vi "Making a Dark Sky Forecast Request.vi"() -> ()   [LabVIEW 2017, in "Dark Sky Weather Data for LabVIEW.lvlib"]
doc: "Example shows how to make a Forecast request to the DarkSky API and inteprets the result. A Forecast request returns the current weather conditions, a minute-by-minute forecast for the next hour (where available), an hour-by-hour forecast for the next 48 hours, and a day-by-day forecast for the next week - all for a given location in latitude and longitude coordinates."
uses:
  Dark Sky Weather Data for LabVIEW.lvlib
  Controls/Units Enum.ctl
  Controls/Language Enum.ctl
panel:
  out "Current Conditions for Request":string
  out "Timezone of Request":string
  in  "Language":T1=enum."English"
  in  "Units":T2="auto"
  in  "Longitude":dbl=-71.0589 min=-180.0 max=180.0
  in  "Latitude":dbl=42.3601 min=-90.0 max=90.0
  in  "API Key":string
  # "Forecast Request"
  # "Powered by Dark Sky"
  # "Required Inputs"
  # "Example Response Subset"
  # "A Forecast request returns the current weather conditions, a minute-by-minute forecast for the next hour (where available), an hour-by-hour forecast for the next 48 hours, and a day-by-day forecast for the next week - all for a given location in latitude and longitude coordinates.\n \nIn order to make a Forecast request, you will need an API key and have already determined the longitude and latitude coordinates of the location you are interested in.\n\nNeed an API Key? Visit: https://darksky.net/dev/ and sign up for free! Enter this API key into the API Key input to run this example."
  # "The Forecast request returns a variety of data. Here is an example where you pull out just the timezone of the requested location along with the summary of current conditions. In this example the default values for latitude and longitude coordinates are for Boston, MA, USA.\n\nVisit https://darksky.net/dev/docs\nfor a complete summary of the data returned by Forecast requests."
  # "Optional Inputs"
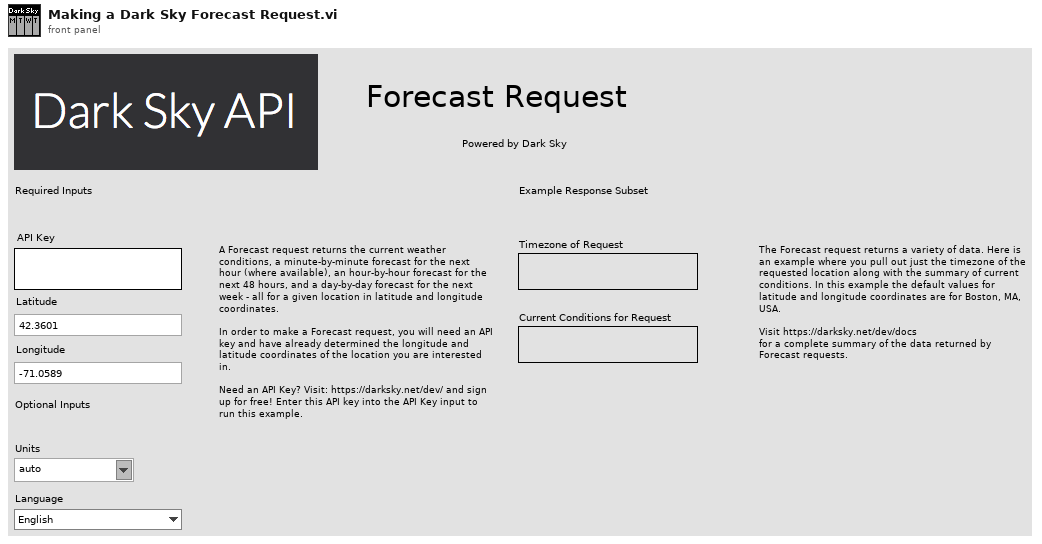
[diagram p1: front panel]
types:
  T1 = typedef "Dark Sky Weather Data for LabVIEW.lvlib/Language Enum.ctl" = enum16{"Arabic", "Azerbaijani", "Belaursian", "Bulgarian", "Bosnian", "Catalan", "Czech", "German", "Greek", "English", "Spanish", "Estonian", "French", "Croatian", "Hungarian", "Indonesian", "Italian", "Icelandic", "Georgian", "Cornish", "Norwegian Bokmal", "Dutch", "Polish", "Portuguese", "Russian", "Slovak", "Slovenian", "Serbian", "Swedish", "Tetum", "Turkish", "Ukrainian", "simplified Chinese", "traditional Chinese"}
  T2 = typedef "Dark Sky Weather Data for LabVIEW.lvlib/Units Enum.ctl" = string
  T3 = typedef "Dark Sky Weather Data for LabVIEW.lvlib/Forecast Output.ctl" = cluster{"Lat, Long, Timezone":T4, "Current Data":T5, "Minutely Data":T6, "Hourly Data":T7, "Daily Data":T8, "Alerts":T9}
  T4 = typedef "Dark Sky Weather Data for LabVIEW.lvlib/Lat_Lon_TZ.ctl" = cluster{"latitude":dbl, "longitude":dbl, "timezone":string, "offset":dbl}
  T5 = typedef "Dark Sky Weather Data for LabVIEW.lvlib/Forecast Current Data.ctl" = cluster{"currently":cluster{"time":dbl, "summary":string, "icon":string, "nearestStormDistance":dbl, "precipIntensity":dbl, "PrecipIntensityError":dbl, "precipProbability":dbl, "precipType":string, "temperature":dbl, "apparentTemp":dbl, "dewPoint":dbl, "humidity":dbl, "windSpeed":dbl, "windGust":dbl, "windBearing":dbl, "visibility":dbl, "cloudCover":dbl, "pressure":dbl, "ozone":dbl}}
  T6 = typedef "Dark Sky Weather Data for LabVIEW.lvlib/Forecast Minutely Data.ctl" = cluster{"minutely":cluster{"summary":string, "icon":string, "data":cluster{"time":dbl, "precipIntensity":dbl, "precipIntensityError":dbl, "precipProbability":dbl, "precipType":string}[]}}
  T7 = typedef "Dark Sky Weather Data for LabVIEW.lvlib/Forecast Hourly Data.ctl" = cluster{"hourly":cluster{"summary":string, "icon":string, "data":cluster{"time":dbl, "summary":string, "icon":string, "precipIntensity":dbl, "precipProbability":dbl, "precipType":string, "temperature":dbl, "apparentTemp":dbl, "dewPoint":dbl, "humidity":dbl, "windSpeed":dbl, "windGust":dbl, "windBearing":dbl, "visibility":dbl, "cloudCover":dbl, "pressure":dbl, "ozone":dbl}[]}}
  T8 = typedef "Dark Sky Weather Data for LabVIEW.lvlib/Forecast Daily Data.ctl" = cluster{"daily":cluster{"summary":string, "icon":string, "data":cluster{"time":dbl, "summary":string, "icon":string, "sunriseTime":dbl, "sunsetTime":dbl, "moonPhase":dbl, "precipIntensity":dbl, "precipIntensityMax":dbl, "precipIntensityMaxTime":dbl, "precipProbability":dbl, "precipType":string, "temperatureMin":dbl, "temperatureMinTime":dbl, "temperatureMax":dbl, "temperatureMaxTime":dbl, "apparentTempMin":dbl, "apparentTempMinTime":dbl, "apparentTempMax":dbl, "apparentTempMaxTime2":dbl, "dewPoint":dbl, "humidity":dbl, "windSpeed":dbl, "windBearing":dbl, "visibility":dbl, "cloudCover":dbl, "pressure":dbl, "ozone":dbl}[]}}
  T9 = typedef "Dark Sky Weather Data for LabVIEW.lvlib/Forecast Alert Data.ctl" = cluster{"alerts":cluster{"title":string, "time":dbl, "expires":dbl, "description":string, "uri":string}[]}
  T10 = cluster{"time":dbl, "summary":string, "icon":string, "nearestStormDistance":dbl, "precipIntensity":dbl, "PrecipIntensityError":dbl, "precipProbability":dbl, "precipType":string, "temperature":dbl, "apparentTemp":dbl, "dewPoint":dbl, "humidity":dbl, "windSpeed":dbl, "windGust":dbl, "windBearing":dbl, "visibility":dbl, "cloudCover":dbl, "pressure":dbl, "ozone":dbl}
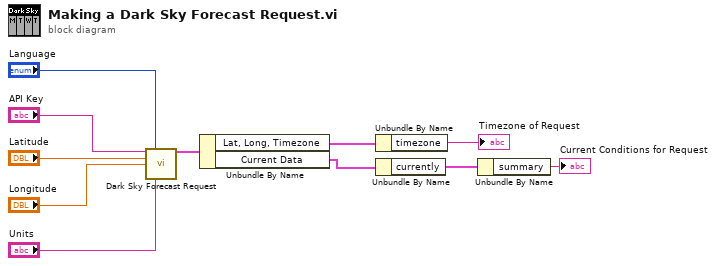
[diagram p0: block diagram]
diagram:
  n1 = call "Dark Sky Forecast Request.vi"("API Key"="API Key", "Language"="Language", "Latitude"="Latitude", "Longitude"="Longitude", "Units"="Units") -> ("Forecast Output"=w6:T3)  [unwired: 9 in, 1 out]
  n2 = Unbundle By Name(w6) -> ("Lat, Long, Timezone"=w5:T4, "Current Data"=w4:T5)
  n3 = Unbundle By Name(w5) -> ("timezone"=→"Timezone of Request":string)
  n4 = Unbundle By Name(w4) -> ("currently"=w3:T10)
  n5 = Unbundle By Name(w3) -> ("summary"=→"Current Conditions for Request":string)
